vi "CFTS-Get CFTS Run Mode.vi"(8 "error in (no error)":errorcluster) -> (0 "error out":errorcluster, 3 "EPL Internal?":bool)   [LabVIEW 2020]
uses:
  <vilib>/Utility/config.llb/Read Key (I32).vi
  <vilib>/Utility/config.llb/NI_LVConfig.lvlib
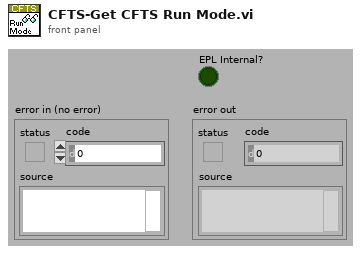
[diagram p1: front panel]
types:
  T1 = typedef "NI_LVConfig.lvlib/Config Data RefNum.ctl" = refnum<k1>
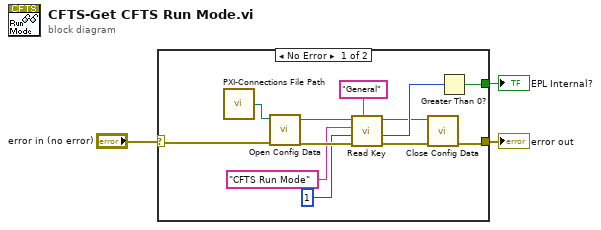
[diagram p0: block diagram]
diagram:
  n1 = case shown="No Error" "error in (no error)" {
    selector: "error in (no error)" -> [w15 w16]
    tunnel: [w10 w16] -> w3
    tunnel: [w6 _] -> w1
    frame No Error {
      n2 = call "PXI-Connections File Path.vi"() -> ("Path"=w4:path)  [unwired: 1 in]
      n3 = call <vilib>:"Open Config Data.vi"("error in (no error)"=w15, "configuration file path"=w4) -> ("error out"=w14:errorcluster, "refnum"=w13:T1)  [unwired: 7 in, 1 out]
      n4 = call-poly <vilib>:"Read Key.vi"("section"="General", "error in (no error)"=w14, "default value"=1, "key"="CFTS Run Mode", "refnum"=w13) -> ("error out"=w8:errorcluster, "value"=w9:i32, "refnum out"=w5:T1)  [unwired: 3 in, 1 out]
      n5 = call <vilib>:"Close Config Data.vi"("error in (no error)"=w8, "refnum"=w5) -> ("error out"=w10:errorcluster)  [unwired: 8 in, 1 out]
      n6 = Greater Than 0?(x=w9) -> (x > 0?=w6:bool)
    }
    frame Error {
    }
  }
  "error out" <- w3
  "EPL Internal?" <- w1
